vi "CDBToString(cast).vi"(1 "输入（CSG)":cdb) -> (0 "字符串（HEX)":string)   [LabVIEW 2012]
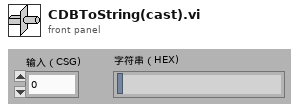
[diagram p1: front panel]
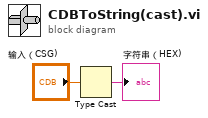
[diagram p0: block diagram]
diagram:
  n1 = Type Cast(x="输入（CSG)") -> (*(type *) &x=→"字符串（HEX)":string)  [unwired: 1 in]
